vi "F Dwf Analog IO Channel Node Get.vi"(7 "pvalue":dbl, 8 "error in (no error)":errorcluster, 9 "idxNode":i32, 10 "idxChannel":i32, 11 "hdwf":i32) -> (0 "error out":errorcluster, 3 "function return":i32, 5 "pvalue out":dbl)   [LabVIEW 2021, in "Olasdwf.lvlib"]
doc: "DWFAPI int FDwfAnalogIOChannelNodeGet(HDWF hdwf, int idxChannel, int idxNode, double *pvalue);"
uses:
  Olasdwf.lvlib
  Windows/System32/dwf.dll
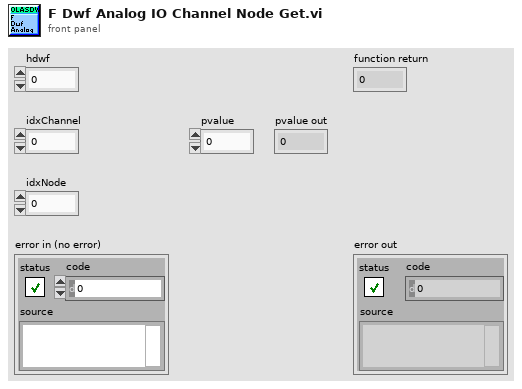
[diagram p1: front panel]
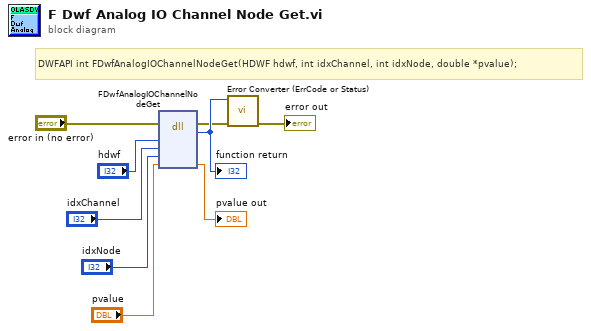
[diagram p0: block diagram]
diagram:
  # "DWFAPI int FDwfAnalogIOChannelNodeGet(HDWF hdwf, int idxChannel, int idxNode, double *pvalue);"
  n1 = dll-call lib="/Windows/System32/dwf.*" fn="FDwfAnalogIOChannelNodeGet"(error in="error in (no error)", "hdwf"="hdwf", "idxChannel"="idxChannel", "idxNode"="idxNode", "pvalue"="pvalue") -> (error out=w2:errorcluster, w9:i32, "pvalue"=→"pvalue out":dbl)  [unwired: 5 in, 1 out]
  "function return" <- w9
  n2 = call "Error Converter (ErrCode or Status).vi"("error in (no error)"=w2, "error code"=w9) -> ("error out"=→"error out":errorcluster)  [unwired: 9 in]
